vi "Check Power Stable.vi"(8 "error in (no error)":errorcluster, 10 "Set Point (mW)":dbl, 11 "LQ Laser in":refnum<class "LQ Laser.lvclass">) -> (0 "error out":errorcluster, 3 "LQ Laser out":refnum<class "LQ Laser.lvclass">)   [LabVIEW 2023, in "LQ Laser.lvlib" / "LQ Laser.lvclass"]
uses:
  LQ Laser.lvclass
  C:/Program Files/National Instruments/LabVIEW 2023/vi.lib/ActorFramework/Actor/Actor.lvclass
  LQ Laser.lvclass/LQ Laser.ctl
  <vilib>/ActorFramework/Actor/Actor.lvclass/Actor.ctl
  <vilib>/ActorFramework/Message Enqueuer/Message Enqueuer.lvclass/Message Enqueuer.ctl
  LQ Laser Messages/Check Power Stable Msg/Check Power Stable Msg.lvclass/Check Power Stable Msg.ctl
  <vilib>/ActorFramework/Message Enqueuer/Init from Existing Queue.vi
  <vilib>/ActorFramework/Message Enqueuer/Enqueue.vi
  LQ Laser Messages/Check Power Stable Msg/Check Power Stable Msg.lvclass
  C:/Program Files/National Instruments/LabVIEW 2023/vi.lib/ActorFramework/Message/Message.lvclass
  Application Messages/Set Laser Power Reply Msg/Set Laser Power Reply Msg.lvclass
  <vilib>/ActorFramework/Message Priority Queue/Priority Enqueue.vi
  <vilib>/ActorFramework/Message Enqueuer/Message Enqueuer.lvclass
  <vilib>/ActorFramework/Actor/Actor.lvclass
panel:
  out "Measured Power":dbl
  out "Response":string
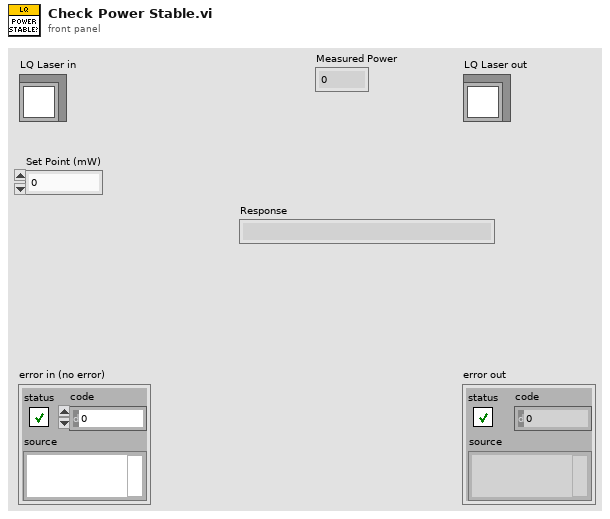
[diagram p1: front panel]
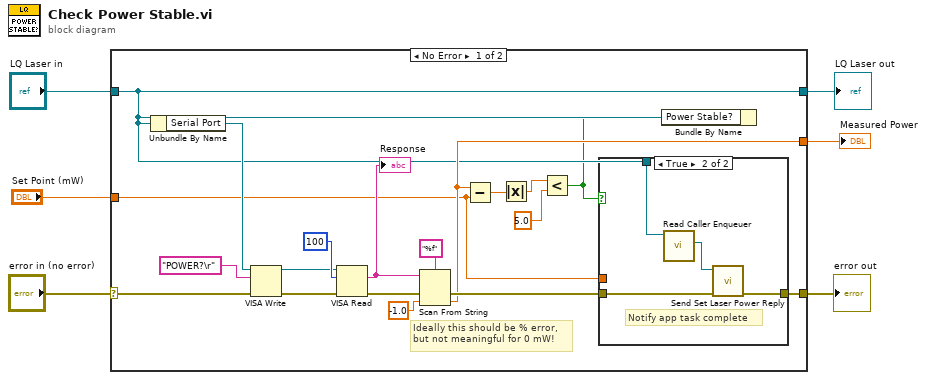
[diagram p0: block diagram]
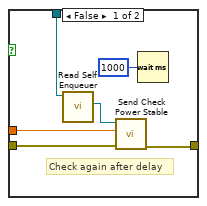
[diagram p2: hidden frame]
diagram:
  n1 = case shown="No Error" "error in (no error)" {
    selector: "error in (no error)" -> [w25 w37]
    tunnel: [w14 w37] -> w3
    tunnel: "LQ Laser in" -> [w11 w36]
    tunnel: [w11 w36] -> w5
    tunnel: "Set Point (mW)" -> [w12 _]
    tunnel: [w13 _] -> w1
    frame No Error {
      # "Ideally this should be % error,\nbut not meaningful for 0 mW!"
      n2 = Unbundle By Name(w11) -> ("Serial Port"=w24:refnum<visa-resource-name>)
      n3 = VISA Write(VISA resource name=w24, write buffer="POWER?\r", error in (no error)=w25) -> (VISA resource name out=w21:refnum<visa-resource-name>, error out=w22:errorcluster)  [unwired: 1 out]
      n4 = VISA Read(VISA resource name=w21, byte count=u32 100, error in (no error)=w22) -> (read buffer=w19:string, error out=w18:errorcluster)  [unwired: 2 out]
      "Response" <- w19
      n5 = Scan From String(format string="%f", input string=w19, error in=w18, default 1=-1.0 ("default value 1")) -> (error out=w15:errorcluster, output 1=w13:dbl)  [unwired: 1 in, 2 out]
      n6 = Subtract(x=w13, y=w12) -> (x-y=w10:dbl)
      n7 = Absolute Value(x=w10) -> (abs(x)=w9:dbl)
      n8 = Less?(x=w9, y=5.0 ("upper limit")) -> (x < y?=w7:bool)
      n9 = case shown="True" w7 {
        tunnel: w15 -> [w29 w35]
        tunnel: [w28 w34] -> w14
        tunnel: w12 -> [w30 _]
        tunnel: w11 -> [w27 w33]
        frame False {
          # "Check again after delay"
          n10 = call <vilib>:"Read Self Enqueuer.vi"("Actor"=w27) -> ("Self Enqueuer"=w26:refnum<class "Message Enqueuer.lvclass">)  [unwired: 10 in]
          n11 = call "Send Check Power Stable.vi"("error in (no error)"=w29, "Set Point (mW)"=w30, "Message Enqueuer"=w26) -> ("error out"=w28:errorcluster)  [unwired: 7 in, 1 out]
          n12 = Wait (ms)(milliseconds to wait=u32 1000) -> ()  [unwired: 1 out]
        }
        frame True {
          # "Notify app task complete"
          n13 = call <vilib>:"Read Caller Enqueuer.vi"("Actor"=w33) -> ("Caller Enqueuer"=w32:refnum<class "Message Enqueuer.lvclass">)  [unwired: 10 in]
          n14 = call "Send Set Laser Power Reply.vi"("error in (no error)"=w35, "Message Enqueuer"=w32) -> ("error out"=w34:errorcluster)  [unwired: 8 in, 1 out]
        }
      }
      n15 = Bundle By Name(cluster=w11, "Power Stable?"=w7) -> ()  [unwired: 1 out]
    }
    frame Error {
    }
  }
  "error out" <- w3
  "LQ Laser out" <- w5
  "Measured Power" <- w1
